vi "addObjToPlasmaBot.vi"(5 "deselectedColor":T1={"Red"=0.0, "Green"=1.0, "Blue"=0.0, "Alpha"=1.0}, 7 "homePos_Offset":cluster{"X":dbl, "Y":dbl, "Z":dbl}, 8 "index":i32, 9 "array":T2[](array[typedef]), 10 "3DpictureRefrenceIn":refnum<vi>) -> (0 "errorOut":errorcluster, 2 "addedObject":T2, 3 "addedObjRefrence":refnum<vi>)   [LabVIEW 2015]
uses:
  processedObjectInfo.ctl
  <vilib>/Utility/miscctls.llb/LVRGBAColorTypeDef.ctl
  <vilib>/picture/3D Picture Control/Object/Create Object (name).vi
  <vilib>/picture/3D Picture Control/NI_3D Picture Control.lvlib
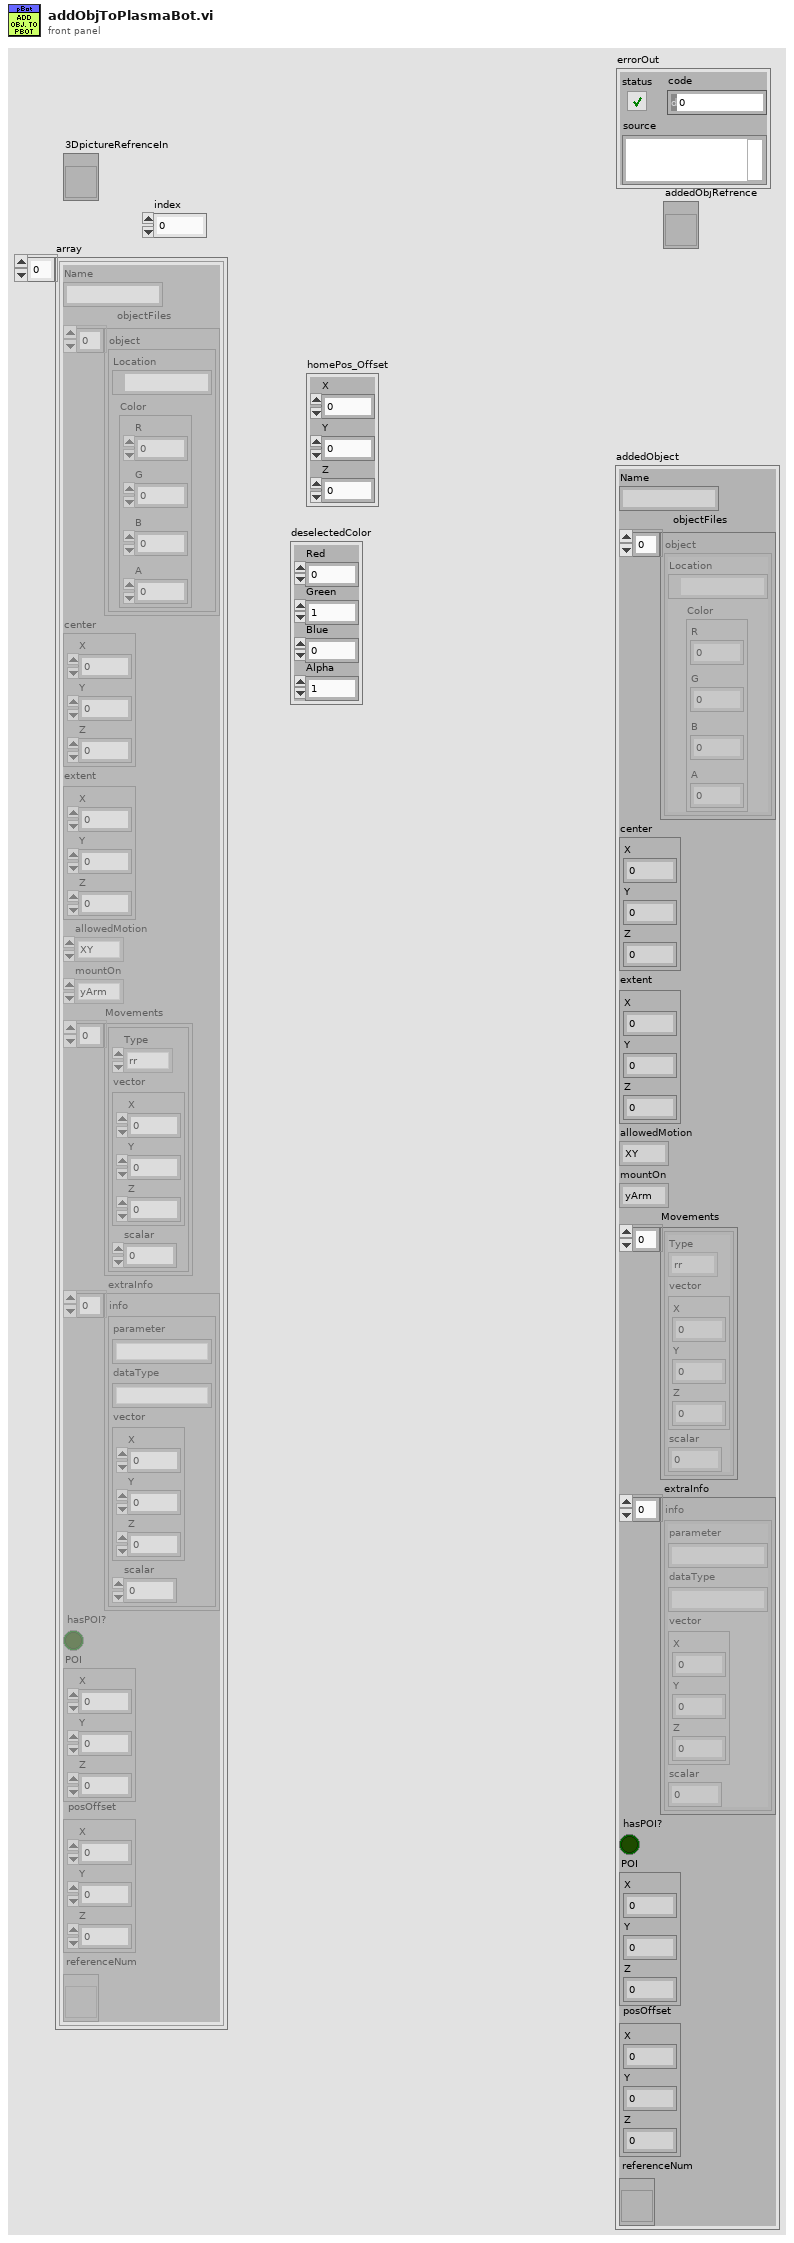
[diagram p1: front panel]
types:
  T1 = typedef "LVRGBAColorTypeDef.ctl" = cluster{"Red":sgl, "Green":sgl, "Blue":sgl, "Alpha":sgl}
  T2 = typedef "processedObjectInfo.ctl" = cluster{"Name":string, "objectFiles":cluster{"Location":path, "Color":cluster{"R":dbl, "G":dbl, "B":dbl, "A":dbl}}[], "center":cluster{"X":dbl, "Y":dbl, "Z":dbl}, "extent":cluster{"X":dbl, "Y":dbl, "Z":dbl}, "allowedMotion":enum16{"XY", "Z"}, "mountOn":enum16{"yArm", "breadBoard"}, "Movements":cluster{"Type":enum16{"rr", "ra", "tr", "ta"}, "vector":cluster{"X":dbl, "Y":dbl, "Z":dbl}, "scalar":dbl}[], "extraInfo":cluster{"parameter":string, "dataType":string, "vector":cluster{"X":dbl, "Y":dbl, "Z":dbl}, "scalar":dbl}[], "hasPOI?":bool, "POI":cluster{"X":dbl, "Y":dbl, "Z":dbl}, "posOffset":cluster{"X":dbl, "Y":dbl, "Z":dbl}, "referenceNum":refnum<vi>}
  T3 = enum16{"Inherit Value", "Points", "Wireframe", "Polygons"}
  T4 = cluster{"Location":path, "Color":cluster{"R":dbl, "G":dbl, "B":dbl, "A":dbl}}[]
  T5 = cluster{"Type":enum16{"rr", "ra", "tr", "ta"}, "vector":cluster{"X":dbl, "Y":dbl, "Z":dbl}, "scalar":dbl}[]
  T6 = cluster{"parameter":string, "dataType":string, "vector":cluster{"X":dbl, "Y":dbl, "Z":dbl}, "scalar":dbl}[]
  T7 = cluster{"Red":sgl, "Green":sgl, "Blue":sgl, "Alpha":sgl}
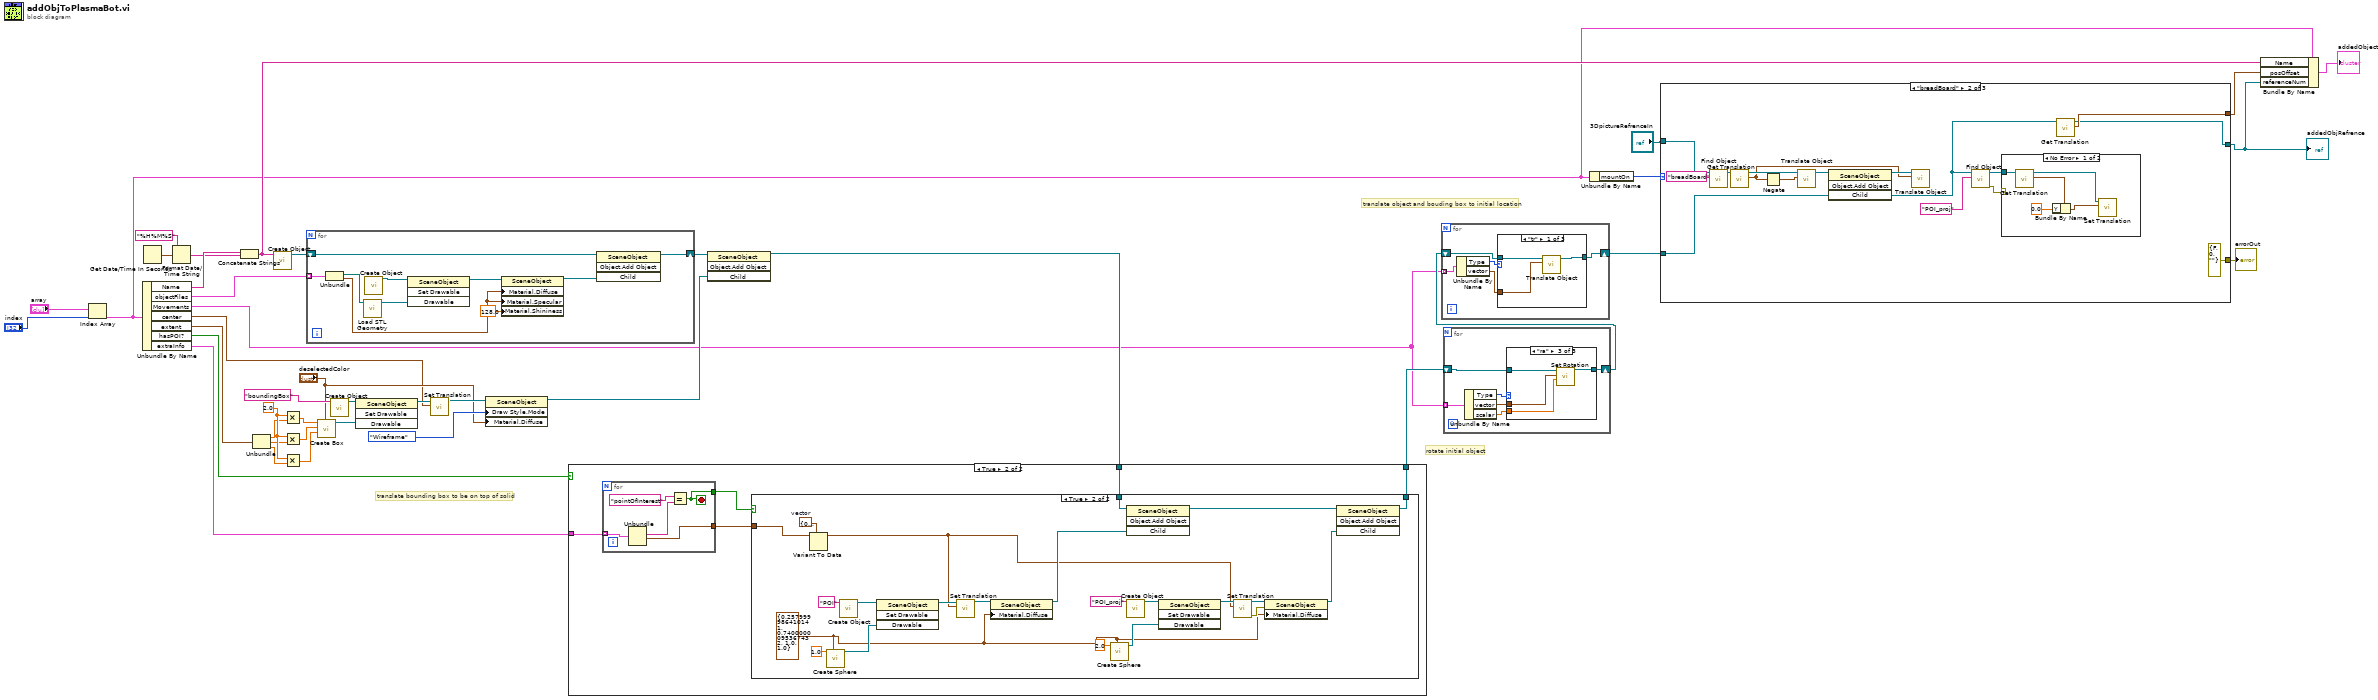
[diagram p0: block diagram]
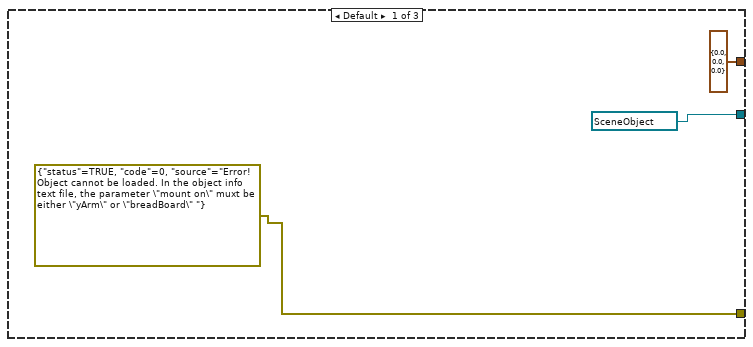
[diagram p4: hidden frame]
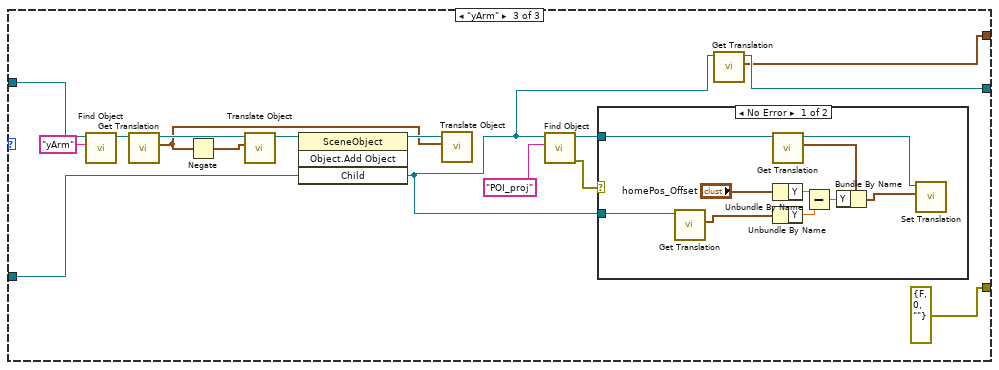
[diagram p6: hidden frame]
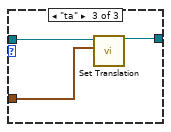
[diagram p9: hidden frame]
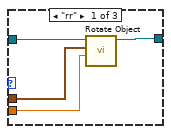
[diagram p10: hidden frame]
diagram:
  w23 = 2.0 ("y")
  # "translate bounding box to be on top of solid"
  # "rotate initial object"
  # "translate object and bouding box to initial location"
  n1 = Index Array(array="array", index="index") -> (element=w9:T2)
  n2 = Unbundle By Name(w9) -> ("Name"=w29:string, "objectFiles"=w3:T4, "Movements"=w2:T5, "center"=w10:cluster{"X":dbl, "Y":dbl, "Z":dbl}, "extent"=w19:cluster{"X":dbl, "Y":dbl, "Z":dbl}, "hasPOI?"=w14:bool, "extraInfo"=w13:T6)
  n3 = Get Date/Time In Seconds() -> (seconds since 1Jan1904=w27:timestamp)
  n4 = Format Date/Time String(time format string (%c)="%H%M%S", seconds (now)=w27) -> (date/time string=w25:string)  [unwired: 1 in]
  n5 = Concatenate Strings(w29, w25) -> (w28:string)
  n6 = Unbundle(w19) -> ("X"=w22:dbl, "Y"=w21:dbl, "Z"=w20:dbl)
  n7 = call-poly <vilib>:"Create Object.vi"("Name"=w28) -> ("Scene:New Object"=w5:refnum<vi>)  [unwired: 9 in, 1 out]
  n8 = Multiply(x=w23, y=w22) -> (x*y=w36:dbl)
  n9 = Multiply(x=w23, y=w21) -> (x*y=w35:dbl)
  n10 = Multiply(x=w23, y=w20) -> (x*y=w34:dbl)
  n11 = for {
    tunnel: w3 -> [w51] mode=indexing
    shift-right: [w44] -> w4
    shift-left: w5 -> [w45]
    n12 = Unbundle(w51) -> ("Location"=w48:path, "Color"=w46:cluster{"R":dbl, "G":dbl, "B":dbl, "A":dbl})
    n13 = call <vilib>:"Load STL Geometry.vi"("Model File"=w48) -> ("New Mesh Refnum"=w49:refnum<vi>)  [unwired: 9 in, 1 out]
    n14 = call-poly <vilib>:"Create Object.vi"() -> ("Scene:New Object"=w50:refnum<vi>)  [unwired: 10 in, 1 out]
    n15 = invoke class="SceneObject" method="Set Drawable"(reference=w50, "Drawable"=w49) -> (reference out=w47:refnum<vi>)  [unwired: 2 in, 3 out]
    n16 = property class="SceneObject"(reference=w47, "Material.Diffuse"=w46, "Material.Specular"=w46, "Material.Shininess"=sgl 128.0 ("Material:Shininess")) -> (reference out=w43:refnum<vi>)  [unwired: 1 in, 1 out]
    n17 = invoke class="SceneObject" method="Object.Add Object"(reference=w45, "Child"=w43) -> (reference out=w44:refnum<vi>)  [unwired: 2 in, 3 out]
  }
  n18 = call <vilib>:"Create Box.vi"("Color"="deselectedColor", "Length Z"=w34, "Length Y"=w35, "Length X"=w36) -> ("New Box Refnum"=w40:refnum<vi>)  [unwired: 6 in, 1 out]
  n19 = call-poly <vilib>:"Create Object.vi"("Name"="boundingBox") -> ("Scene:New Object"=w41:refnum<vi>)  [unwired: 9 in, 1 out]
  n20 = invoke class="SceneObject" method="Set Drawable"(reference=w41, "Drawable"=w40) -> (reference out=w39:refnum<vi>)  [unwired: 2 in, 3 out]
  n21 = call <vilib>:"Set Translation.vi"("Translation"=w10, "Scene Object"=w39) -> ("Translated Object"=w37:refnum<vi>)  [unwired: 8 in, 1 out]
  n22 = property class="SceneObject"(reference=w37, "Draw Style.Mode"=T3."Wireframe" ("Draw Style:Mode"), "Material.Diffuse"="deselectedColor") -> (reference out=w33:refnum<vi>)  [unwired: 1 in, 1 out]
  n23 = invoke class="SceneObject" method="Object.Add Object"(reference=w4, "Child"=w33) -> (reference out=w12:refnum<vi>)  [unwired: 2 in, 3 out]
  n24 = case shown="True" w14 {
    tunnel: w13 -> [_ w57]
    tunnel: w12 -> [w52 w56]
    tunnel: [w52 w55] -> w11
    frame False {
    }
    frame True {
      n25 = for {
        tunnel: w57 -> [w85] mode=indexing
        tunnel: [w81] -> w53
        tunnel: [w82] -> w54
        stop <- w82 stop-if-true
        n26 = Unbundle(w85) -> ("dataType"=w83:string, "vector"=w81:cluster{"X":dbl, "Y":dbl, "Z":dbl})  [unwired: 2 out]
        n27 = Equal?(x="pointOfInterest" ("Name"), y=w83) -> (x = y?=w82:bool)
      }
      n28 = case shown="True" w54 {
        tunnel: w56 -> [w58 w72]
        tunnel: [w58 w70] -> w55
        tunnel: w53 -> [_ w69]
        frame False {
        }
        frame True {
          w68 = cluster{"X":dbl, "Y":dbl, "Z":dbl} {"X"=0.0, "Y"=0.0, "Z"=0.0}  # vector
          w62 = T7 {"Red"=0.258, "Green"=0.74, "Blue"=1.0, "Alpha"=1.0} ("Color")
          n29 = Variant To Data(type=w68, Variant=w69) -> (data=w60:cluster{"X":dbl, "Y":dbl, "Z":dbl})  [unwired: 1 in, 1 out]
          n30 = call <vilib>:"Create Sphere.vi"("Color"=w62, "Radius"=sgl 1.0) -> ("New Sphere Refnum"=w75:refnum<vi>)  [unwired: 8 in, 1 out]
          n31 = call-poly <vilib>:"Create Object.vi"("Name"="POI") -> ("Scene:New Object"=w77:refnum<vi>)  [unwired: 9 in, 1 out]
          n32 = invoke class="SceneObject" method="Set Drawable"(reference=w77, "Drawable"=w75) -> (reference out=w74:refnum<vi>)  [unwired: 2 in, 3 out]
          n33 = call <vilib>:"Set Translation.vi"("Translation"=w60, "Scene Object"=w74) -> ("Translated Object"=w63:refnum<vi>)  [unwired: 8 in, 1 out]
          n34 = property class="SceneObject"(reference=w63, "Material.Diffuse"=w62) -> (reference out=w61:refnum<vi>)  [unwired: 1 in, 1 out]
          n35 = call <vilib>:"Create Sphere.vi"("Color"=w62, "Radius"=sgl 2.0) -> ("New Sphere Refnum"=w66:refnum<vi>)  [unwired: 8 in, 1 out]
          n36 = invoke class="SceneObject" method="Object.Add Object"(reference=w72, "Child"=w61) -> (reference out=w71:refnum<vi>)  [unwired: 2 in, 3 out]
          n37 = call-poly <vilib>:"Create Object.vi"("Name"="POI_proj") -> ("Scene:New Object"=w76:refnum<vi>)  [unwired: 9 in, 1 out]
          n38 = invoke class="SceneObject" method="Set Drawable"(reference=w76, "Drawable"=w66) -> (reference out=w73:refnum<vi>)  [unwired: 2 in, 3 out]
          n39 = call <vilib>:"Set Translation.vi"("Translation"=w60, "Scene Object"=w73) -> ("error out"=w64:errorcluster, "Translated Object"=w65:refnum<vi>)  [unwired: 8 in]
          n40 = property class="SceneObject"(reference=w65, error in=w64, "Material.Diffuse"=w62) -> (reference out=w59:refnum<vi>)  [unwired: 1 out]
          n41 = invoke class="SceneObject" method="Object.Add Object"(reference=w71, "Child"=w59) -> (reference out=w70:refnum<vi>)  [unwired: 2 in, 3 out]
        }
      }
    }
  }
  n42 = for {
    tunnel: w2 -> [w91] mode=indexing
    shift-right: [w86] -> w18
    shift-left: w11 -> [w87]
    n43 = Unbundle By Name(w91) -> ("Type"=w90:enum16{"rr", "ra", "tr", "ta"}, "vector"=w89:cluster{"X":dbl, "Y":dbl, "Z":dbl}, "scalar"=w88:dbl)
    n44 = case shown="\"ra\"" w90 {
      tunnel: w89 -> [w92 _ w98]
      tunnel: w88 -> [w93 _ w97]
      tunnel: w87 -> [w95 w96 w100]
      tunnel: [w94 w96 w99] -> w86
      frame "rr" {
        n45 = call <vilib>:"Rotate Object.vi"("Angle"=w93, "Axis"=w92, "Scene.Object In"=w95) -> ("Scene.Object Out"=w94:refnum<vi>)  [unwired: 7 in, 1 out]
      }
      frame Default {
      }
      frame "ra" {
        n46 = call <vilib>:"Set Rotation.vi"("Angle"=w97, "Axis"=w98, "Scene Object"=w100) -> ("Rotated Scene Object"=w99:refnum<vi>)  [unwired: 7 in, 1 out]
      }
    }
  }
  n47 = for {
    tunnel: w2 -> [w105] mode=indexing
    shift-right: [w101] -> w17
    shift-left: w18 -> [w104]
    n48 = Unbundle By Name(w105) -> ("Type"=w103:enum16{"rr", "ra", "tr", "ta"}, "vector"=w102:cluster{"X":dbl, "Y":dbl, "Z":dbl})
    n49 = case shown="\"tr\"" w103 {
      tunnel: w102 -> [w106 _ w110]
      tunnel: w104 -> [w108 w109 w112]
      tunnel: [w107 w109 w111] -> w101
      frame "tr" {
        n50 = call <vilib>:"Translate Object.vi"("Translation"=w106, "Scene.Object In"=w108) -> ("Scene.Object Out"=w107:refnum<vi>)  [unwired: 8 in, 1 out]
      }
      frame Default {
      }
      frame "ta" {
        n51 = call <vilib>:"Set Translation.vi"("Translation"=w110, "Scene Object"=w112) -> ("Translated Object"=w111:refnum<vi>)  [unwired: 8 in, 1 out]
      }
    }
  }
  n52 = Unbundle By Name(w9) -> ("mountOn"=w1:enum16{"yArm", "breadBoard"})
  n53 = case shown="\"breadBoard\"" w1 {
    tunnel: w17 -> [_ w125 w146]
    tunnel: [refnum<vi> refnum ("Scene.Object Out") w118 w140] -> w7
    tunnel: "3DpictureRefrenceIn" -> [_ w131 w152]
    tunnel: [cluster{"X":sgl, "Y":sgl, "Z":sgl} {"X"=0.0, "Y"=0.0, "Z"=0.0} ("Transformation:Get Translation") w119 w139] -> w8
    tunnel: [errorcluster {"status"=TRUE, "code"=0, "source"="Error! Object cannot be loaded. In the object info text file, the parameter \"mount on\" muxt be either \"yArm\" or \"breadBoard\" "} ("error constant") errorcluster {"status"=FALSE, "code"=0, "source"=""} ("error constant") errorcluster {"status"=FALSE, "code"=0, "source"=""} ("error constant")] -> w6
    frame Default {
    }
    frame "breadBoard" {
      n54 = call <vilib>:"Find Object.vi"("Object Name"="breadBoard", "Scene Refnum"=w131) -> ("Object Refnum"=w130:refnum<vi>)  [unwired: 8 in, 1 out]
      n55 = call <vilib>:"Get Translation.vi"("Scene Object"=w130) -> ("Transformation:Get Translation"=w121:cluster{"X":sgl, "Y":sgl, "Z":sgl}, "Scene Object"=w129:refnum<vi>)  [unwired: 8 in, 1 out]
      n56 = Negate(x=w121) -> (-x=w126:cluster{"X":sgl, "Y":sgl, "Z":sgl})
      n57 = call <vilib>:"Translate Object.vi"("Translation"=w126, "Scene.Object In"=w129) -> ("Scene.Object Out"=w128:refnum<vi>)  [unwired: 8 in, 1 out]
      n58 = invoke class="SceneObject" method="Object.Add Object"(reference=w128, "Child"=w125) -> (reference out=w127:refnum<vi>, "Child"=w120:refnum<vi>)  [unwired: 2 in, 2 out]
      n59 = call <vilib>:"Translate Object.vi"("Translation"=w121, "Scene.Object In"=w127) -> ()  [unwired: 8 in, 2 out]
      n60 = call <vilib>:"Find Object.vi"("Object Name"="POI_proj", "Scene Refnum"=w120) -> ("error out"=w122:errorcluster, "Object Refnum"=w123:refnum<vi>)  [unwired: 8 in]
      n61 = case shown="No Error" w122 {
        tunnel: w123 -> [w136 _]
        frame No Error {
          n62 = call <vilib>:"Get Translation.vi"("Scene Object"=w136) -> ("Transformation:Get Translation"=w135:cluster{"X":sgl, "Y":sgl, "Z":sgl}, "Scene Object"=w134:refnum<vi>)  [unwired: 8 in, 1 out]
          n63 = Bundle By Name(cluster=w135, "Y"=sgl 0.0) -> (w133:cluster{"X":sgl, "Y":sgl, "Z":sgl})
          n64 = call <vilib>:"Set Translation.vi"("Translation"=w133, "Scene Object"=w134) -> ()  [unwired: 8 in, 2 out]
        }
        frame Error {
        }
      }
      n65 = call <vilib>:"Get Translation.vi"("Scene Object"=w120) -> ("Transformation:Get Translation"=w119:cluster{"X":sgl, "Y":sgl, "Z":sgl}, "Scene Object"=w118:refnum<vi>)  [unwired: 8 in, 1 out]
    }
    frame "yArm" {
      n66 = call <vilib>:"Find Object.vi"("Object Name"="yArm", "Scene Refnum"=w152) -> ("Object Refnum"=w151:refnum<vi>)  [unwired: 8 in, 1 out]
      n67 = call <vilib>:"Get Translation.vi"("Scene Object"=w151) -> ("Transformation:Get Translation"=w142:cluster{"X":sgl, "Y":sgl, "Z":sgl}, "Scene Object"=w150:refnum<vi>)  [unwired: 8 in, 1 out]
      n68 = Negate(x=w142) -> (-x=w147:cluster{"X":sgl, "Y":sgl, "Z":sgl})
      n69 = call <vilib>:"Translate Object.vi"("Translation"=w147, "Scene.Object In"=w150) -> ("Scene.Object Out"=w149:refnum<vi>)  [unwired: 8 in, 1 out]
      n70 = invoke class="SceneObject" method="Object.Add Object"(reference=w149, "Child"=w146) -> (reference out=w148:refnum<vi>, "Child"=w141:refnum<vi>)  [unwired: 2 in, 2 out]
      n71 = call <vilib>:"Translate Object.vi"("Translation"=w142, "Scene.Object In"=w148) -> ()  [unwired: 8 in, 2 out]
      n72 = call <vilib>:"Find Object.vi"("Object Name"="POI_proj", "Scene Refnum"=w141) -> ("error out"=w143:errorcluster, "Object Refnum"=w144:refnum<vi>)  [unwired: 8 in]
      n73 = case shown="No Error" w143 {
        tunnel: w144 -> [w162 _]
        tunnel: w141 -> [w154 _]
        frame No Error {
          n74 = call <vilib>:"Get Translation.vi"("Scene Object"=w154) -> ("Transformation:Get Translation"=w153:cluster{"X":sgl, "Y":sgl, "Z":sgl})  [unwired: 8 in, 2 out]
          n75 = call <vilib>:"Get Translation.vi"("Scene Object"=w162) -> ("Transformation:Get Translation"=w160:cluster{"X":sgl, "Y":sgl, "Z":sgl}, "Scene Object"=w159:refnum<vi>)  [unwired: 8 in, 1 out]
          n76 = Unbundle By Name("homePos_Offset") -> ("Y"=w156:dbl)
          n77 = Unbundle By Name(w153) -> ("Y"=w155:sgl)
          n78 = Subtract(x=w156, y=w155) -> (x-y=w157:dbl)
          n79 = Bundle By Name(cluster=w160, "Y"=w157) -> (w158:cluster{"X":sgl, "Y":sgl, "Z":sgl})
          n80 = call <vilib>:"Set Translation.vi"("Translation"=w158, "Scene Object"=w159) -> ()  [unwired: 8 in, 2 out]
        }
        frame Error {
        }
      }
      n81 = call <vilib>:"Get Translation.vi"("Scene Object"=w141) -> ("Transformation:Get Translation"=w139:cluster{"X":sgl, "Y":sgl, "Z":sgl}, "Scene Object"=w140:refnum<vi>)  [unwired: 8 in, 1 out]
    }
  }
  "addedObjRefrence" <- w7
  "errorOut" <- w6
  n82 = Bundle By Name(cluster=w9, "Name"=w28, "posOffset"=w8, "referenceNum"=w7) -> (→"addedObject":T2)
